vi "Read Attributes.vi"(11 "Send Status String Msg":refnum<class "Status String Msg.lvclass">) -> (2 "Payload":cluster{"Status":string})   [LabVIEW 2017, in "Test.lvlib" / "Status String Msg.lvclass"]
uses:
  Status String Msg.lvclass
  Status String Msg.lvclass/Status String Msg.ctl
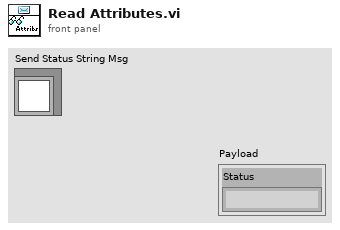
[diagram p1: front panel]
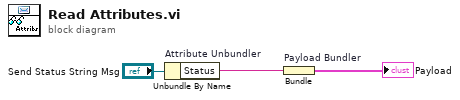
[diagram p0: block diagram]
diagram:
  n1 = Unbundle By Name "Attribute Unbundler"("Send Status String Msg") -> ("Status"=w1:string)
  n2 = Bundle "Payload Bundler"("Status"=w1) -> (→"Payload":cluster{"Status":string})  [unwired: 1 in]
